vi "md5.vi"(11 "Data in":string) -> (2 "MD5 (16-bytes)":string, 3 "MD5 (Hex String)":string)   [LabVIEW 2021, in "hashlib.lvlib"]
doc: "Calculates the md5 checksum.\n\n[RFC 1321]"
uses:
  hashlib.lvlib
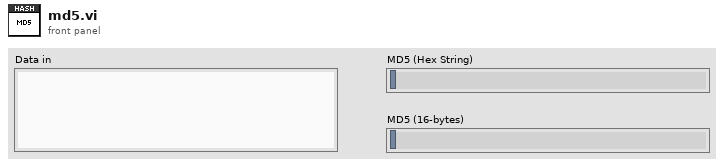
[diagram p1: front panel]
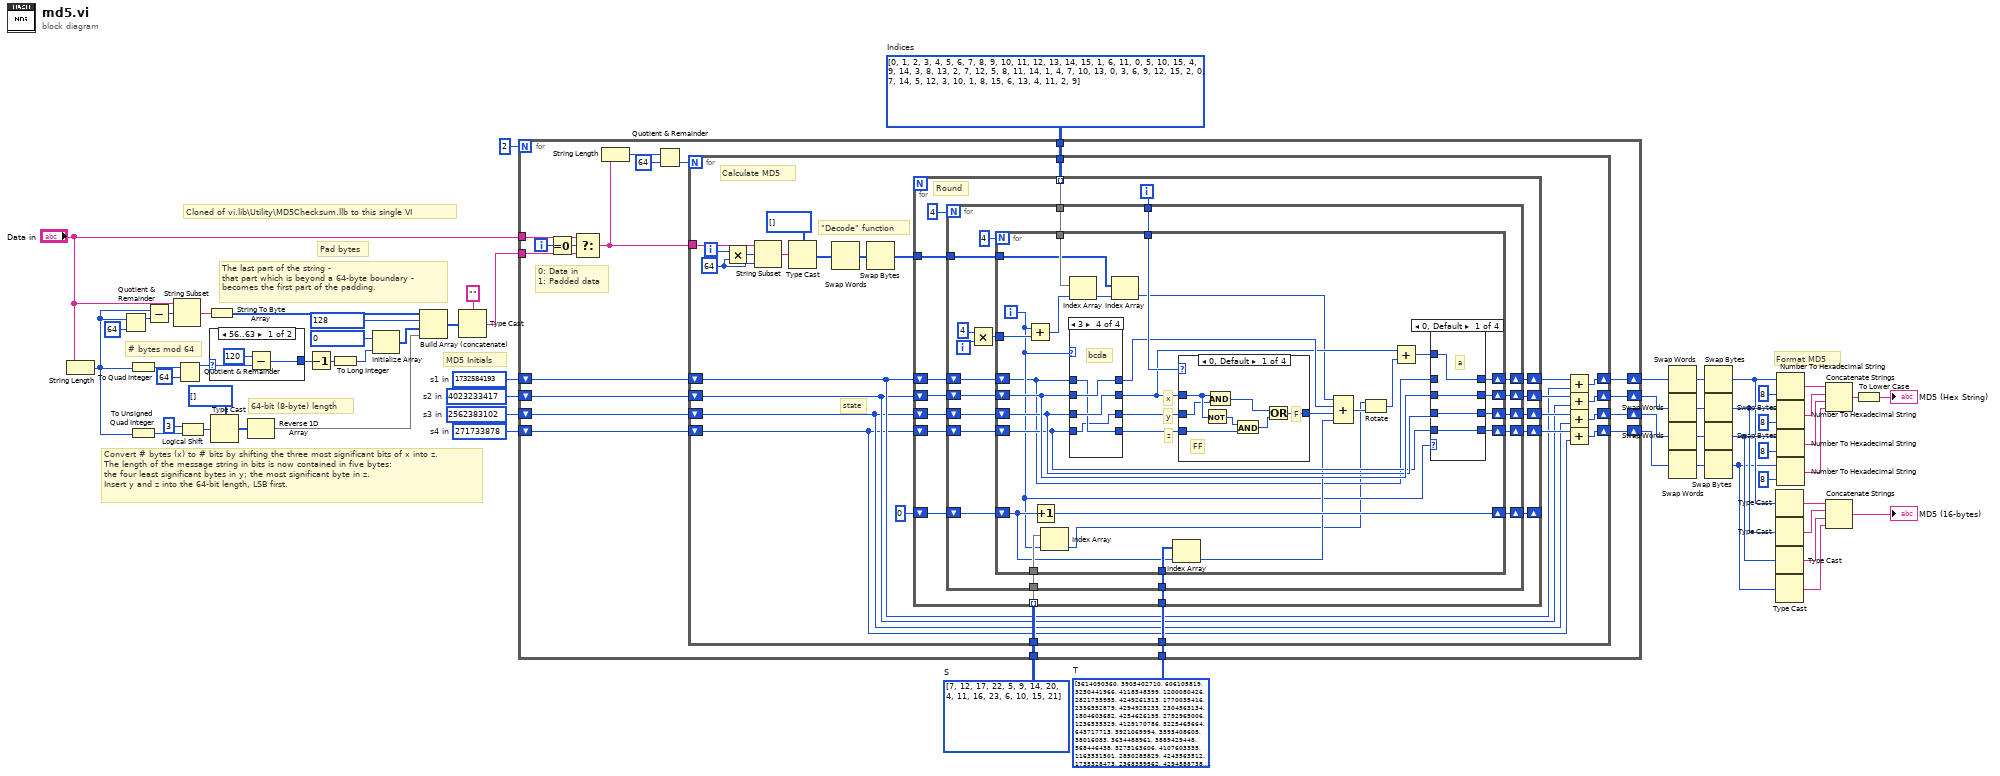
[diagram p0: block diagram]
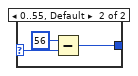
[diagram p2: hidden frame]
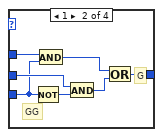
[diagram p3: hidden frame]
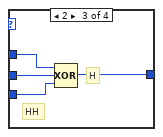
[diagram p4: hidden frame]
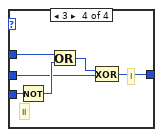
[diagram p5: hidden frame]
diagram:
  w43 = u32 1732584193  # s1 in
  w42 = u32 4023233417  # s2 in
  w41 = u32 2562383102  # s3 in
  w40 = u32 271733878  # s4 in
  w47 = i32[][] [[7, 12, 17, 22], [5, 9, 14, 20], [4, 11, 16, 23], [6, 10, 15, 21]]  # S
  w46 = u32[] [3614090360, 3905402710, 606105819, 3250441966, 4118548399, 1200080426, 2821735955, 4249261313, 1770035416, 2336552879, 4294925233, 2304563134, 1804603682, 4254626195, 2792965006, 1236535329, 4129170786, 3225465664, 643717713, 3921069994, 3593408605, 38016083, 3634488961, 3889429448, 568446438, 3275163606, 4107603335, 1163531501, 2850285829, 4243563512, 1735328473, 2368359562, 4294588738, 2272392833, 1839030562, 4259657740, 2763975236, 1272893353, 4139469664, 3200236656, 681279174, 3936430074, 3572445317, 76029189, 3654602809, 3873151461, 530742520, 3299628645, 4096336452, 1126891415, 2878612391, 4237533241, 1700485571, 2399980690, 4293915773, 2240044497, 1873313359, 4264355552, 2734768916, 1309151649, 4149444226, 3174756917, 718787259, 3951481745]  # T
  w45 = i32[][] [[0, 1, 2, 3, 4, 5, 6, 7, 8, 9, 10, 11, 12, 13, 14, 15], [1, 6, 11, 0, 5, 10, 15, 4, 9, 14, 3, 8, 13, 2, 7, 12], [5, 8, 11, 14, 1, 4, 7, 10, 13, 0, 3, 6, 9, 12, 15, 2], [0, 7, 14, 5, 12, 3, 10, 1, 8, 15, 6, 13, 4, 11, 2, 9]]  # Indices
  # "Cloned of vi.lib\\Utility\\MD5Checksum.llb to this single VI"
  # "Format MD5"
  # "MD5 Initials"
  # "Pad bytes"
  # "The last part of the string - \nthat part which is beyond a 64-byte boundary - \nbecomes the first part of the padding."
  # "64-bit (8-byte) length"
  # "Convert # bytes (x) to # bits by shifting the three most significant bits of x into z.\nThe length of the message string in bits is now contained in five bytes:  \nthe four least significant bytes in y; the most significant byte in z.\nInsert y and z into the 64-bit length, LSB first."
  # "# bytes mod 64"
  n1 = String Length(string="Data in") -> (length=w58:i32)
  n2 = Quotient & Remainder(x=w58, y=64) -> (x-y*floor(x/y)=w57:i32)  [unwired: 1 out]
  n3 = To Quad Integer(1:w58) -> (0:w24:i64)
  n4 = To Unsigned Quad Integer(1:w58) -> (0:w35:u64)
  n5 = Subtract(x=w58, y=w57) -> (x-y=w59:i32)
  n6 = String Subset(string="Data in", offset (0)=w59) -> (substring=w56:string)  [unwired: 1 out]
  n7 = Quotient & Remainder(x=w24, y=i64 64) -> (x-y*floor(x/y)=w33:i64)  [unwired: 1 out]
  n8 = Logical Shift(y=i16 3, x=w35) -> (x << y=w37:u64)
  n9 = String To Byte Array(string=w56) -> (unsigned byte array=w32:u8[])
  n10 = case shown="56..63" w33 {
    selector: w33 -> [w62 w65]
    tunnel: [w61 w64] -> w31
    frame 56..63 {
      n11 = Subtract(x=i64 120, y=w62) -> (x-y=w61:i64)
    }
    frame 0..55, Default {
      n12 = Subtract(x=i64 56, y=w65) -> (x-y=w64:i64)
    }
  }
  n13 = Type Cast(type=u8[] [], x=w37) -> (*(type *) &x=w38:u8[])
  n14 = Reverse 1D Array(array=w38) -> (reversed array=w39:u8[])
  n15 = Decrement(x=w31) -> (x-1=w30:i64)
  n16 = To Long Integer(number=w30) -> (32bit integer=w22:i32)
  n17 = Initialize Array(u8 0, w22) -> (w26:u8[])
  n18 = Build Array (concatenate)(w32, u8 128, w26, w39) -> (w29:u8[])
  n19 = Type Cast(type="", x=w29) -> (*(type *) &x=w52:string)
  n20 = for {
    N: 2 -> [_]
    tunnel: w47 -> [w77]
    tunnel: w46 -> [w76]
    tunnel: w45 -> [w75]
    tunnel: "Data in" -> [w68]
    shift-right: [w78] -> w51
    shift-left: w43 -> [w82]
    shift-right: [w79] -> w50
    shift-left: w42 -> [w83]
    shift-right: [w80] -> w49
    shift-left: w41 -> [w84]
    shift-right: [w81] -> w48
    shift-left: w40 -> [w85]
    tunnel: w52 -> [w67]
    i -> [w71]
    # "0: Data in\n1: Padded data"
    n21 = Equal To 0?(x=w71) -> (x = 0?=w70:bool)
    n22 = Select(t=w68, s=w70, f=w67) -> (s? t:f=w69:string)
    n23 = String Length(string=w69) -> (length=w73:i32)
    n24 = Quotient & Remainder(x=w73, y=64) -> (floor(x/y)=w72:i32)  [unwired: 1 out]
    n25 = for {
      N: w72 -> [_]
      tunnel: w75 -> [w105]
      tunnel: w76 -> [w104]
      tunnel: w77 -> [w103]
      shift-right: [w102] -> w78
      shift-left: w82 -> [w98]
      shift-right: [w101] -> w79
      shift-left: w83 -> [w97]
      shift-right: [w100] -> w80
      shift-left: w84 -> [w96]
      shift-right: [w99] -> w81
      shift-left: w85 -> [w95]
      tunnel: w69 -> [w93]
      i -> [w94]
      w86 = 64 ("y")
      # "Calculate MD5"
      # "\"Decode\" function"
      # "state"
      n26 = Multiply(x=w94, y=w86) -> (x*y=w90:i32)
      n27 = String Subset(string=w93, offset (0)=w90, length (rest)=w86) -> (substring=w92:string)
      n28 = Type Cast(type=u32[] [], x=w92) -> (*(type *) &x=w88:u32[])
      n29 = Swap Words(1:w88) -> (0:w89:u32[])
      n30 = Swap Bytes(anything=w89) -> (byte swapped=w87:u32[])
      n31 = for {
        shift-right: [w121] -> w107
        shift-left: w98 -> [w122]
        shift-right: [w120] -> w108
        shift-left: w97 -> [w123]
        shift-right: [w119] -> w109
        shift-left: w96 -> [w124]
        shift-right: [w118] -> w110
        shift-left: w95 -> [w125]
        tunnel: w105 -> [w117] mode=indexing
        tunnel: w103 -> [w116] mode=indexing
        tunnel: w87 -> [w115]
        shift-right: [w112] -> _
        shift-left: 0 -> [w113]
        tunnel: w104 -> [w111]
        i -> [w126]
        # "Round"
        n32 = for {
          N: 4 -> [_]
          tunnel: w126 -> [w145]
          shift-right: [w138] -> w118
          shift-left: w125 -> [w139]
          shift-right: [w137] -> w119
          shift-left: w124 -> [w140]
          shift-right: [w143] -> w120
          shift-left: w123 -> [w141]
          shift-right: [w144] -> w121
          shift-left: w122 -> [w142]
          tunnel: w117 -> [w136]
          tunnel: w116 -> [w135]
          tunnel: w115 -> [w131]
          shift-right: [w128] -> w112
          shift-left: w113 -> [w129]
          tunnel: w111 -> [w127]
          i -> [w134]
          n33 = Multiply(x=4, y=w134) -> (x*y=w132:i32)
          n34 = for {
            N: 4 -> [_]
            tunnel: w145 -> [w157]
            shift-right: [w167] -> w138
            shift-left: w139 -> [w162]
            shift-right: [w166] -> w137
            shift-left: w140 -> [w163]
            shift-right: [w165] -> w143
            shift-left: w141 -> [w164]
            shift-right: [w168] -> w144
            shift-left: w142 -> [w148]
            tunnel: w136 -> [w175]
            tunnel: w135 -> [w174]
            tunnel: w132 -> [w161]
            tunnel: w131 -> [w171]
            shift-right: [w158] -> w128
            shift-left: w129 -> [w159]
            tunnel: w127 -> [w160]
            i -> [w149]
            # "z"
            # "y"
            # "x"
            n35 = Add(x=w149, y=w161) -> (x+y=w173:i32)
            n36 = Increment(x=w159) -> (x+1=w158:i32)
            n37 = Index Array(array=w174, index=w149) -> (element=w147:i32)
            n38 = Index Array(array=w175, index=w173) -> (element=w172:i32)
            n39 = case shown="3" w149 {
              tunnel: w148 -> [w219 w222 w225 w229]
              tunnel: w164 -> [w218 w221 w224 w231]
              tunnel: w163 -> [w217 w220 w227 w230]
              tunnel: w162 -> [w216 w223 w226 w228]
              tunnel: [w219 w223 w227 w231] -> w152
              tunnel: [w218 w222 w226 w230] -> w151
              tunnel: [w217 w221 w225 w228] -> w170
              tunnel: [w216 w220 w224 w229] -> w169
              frame 0, Default {
                # "abcd"
              }
              frame 1 {
                # "dabc"
              }
              frame 2 {
                # "cdab"
              }
              frame 3 {
                # "bcda"
              }
            }
            n40 = Index Array(array=w171, index=w172) -> (element=w146:u32)
            n41 = Index Array(array=w160, index=w159) -> (element=w154:u32)
            n42 = case shown="0, Default" w157 {
              tunnel: w151 -> [w179 w185 w192 w196]
              tunnel: w170 -> [w178 w184 w193 w195]
              tunnel: w169 -> [w177 w183 w191 w194]
              tunnel: [w176 w186 w190 w197] -> w153
              frame 0, Default {
                # "FF"
                # "F"
                n43 = Not(x=w179) -> (.not. x?=w182:u32)
                n44 = And(x=w179, y=w178) -> (x .and. y?=w181:u32)
                n45 = And(x=w182, y=w177) -> (x .and. y?=w180:u32)
                n46 = Or(x=w181, y=w180) -> (x .or. y?=w176:u32)
              }
              frame 1 {
                # "GG"
                # "G"
                n47 = Not(x=w183) -> (.not. x?=w187:u32)
                n48 = And(x=w185, y=w183) -> (x .and. y?=w188:u32)
                n49 = And(x=w184, y=w187) -> (x .and. y?=w189:u32)
                n50 = Or(x=w188, y=w189) -> (x .or. y?=w186:u32)
              }
              frame 2 {
                # "H"
                # "HH"
                n51 = Compound Arithmetic op=XOR(w192, w193, w191) -> (w190:u32)
              }
              frame 3 {
                # "I"
                # "II"
                n52 = Not(x=w194) -> (.not. x?=w199:u32)
                n53 = Or(x=w196, y=w199) -> (x .or. y?=w198:u32)
                n54 = Exclusive Or(1:w195, 2:w198) -> (0:w197:u32)
              }
            }
            n55 = Compound Arithmetic op=ADD(w146, w152, w153, w154) -> (w156:u32)
            n56 = Rotate(1:w156, 2:w147) -> (0:w150:u32)
            n57 = Add(x=w151, y=w150) -> (x+y=w155:u32)
            n58 = case shown="0, Default" w149 {
              tunnel: w155 -> [w203 w207 w211 w215]
              tunnel: [w203 w206 w210 w214] -> w168
              tunnel: [w200 w207 w208 w212] -> w167
              tunnel: [w201 w204 w211 w213] -> w166
              tunnel: [w202 w205 w209 w215] -> w165
              tunnel: w148 -> [_ w206 w210 w214]
              tunnel: w164 -> [w202 w205 w209 _]
              tunnel: w163 -> [w201 w204 _ w213]
              tunnel: w162 -> [w200 _ w208 w212]
              frame 0, Default {
                # "a"
              }
              frame 1 {
                # "d"
              }
              frame 2 {
                # "c"
              }
              frame 3 {
                # "b"
              }
            }
          }
        }
      }
      n59 = Add(x=w107, y=w98) -> (x+y=w102:u32)
      n60 = Add(x=w108, y=w97) -> (x+y=w101:u32)
      n61 = Add(x=w109, y=w96) -> (x+y=w100:u32)
      n62 = Add(x=w110, y=w95) -> (x+y=w99:u32)
    }
  }
  n63 = Swap Words(1:w51) -> (0:w2:u32)
  n64 = Swap Words(1:w50) -> (0:w3:u32)
  n65 = Swap Words(1:w49) -> (0:w6:u32)
  n66 = Swap Words(1:w48) -> (0:w7:u32)
  n67 = Swap Bytes(anything=w2) -> (byte swapped=w15:u32)
  n68 = Swap Bytes(anything=w3) -> (byte swapped=w16:u32)
  n69 = Swap Bytes(anything=w6) -> (byte swapped=w17:u32)
  n70 = Swap Bytes(anything=w7) -> (byte swapped=w14:u32)
  n71 = Type Cast(x=w15) -> (*(type *) &x=w18:string)  [unwired: 1 in]
  n72 = Type Cast(x=w16) -> (*(type *) &x=w19:string)  [unwired: 1 in]
  n73 = Type Cast(x=w17) -> (*(type *) &x=w20:string)  [unwired: 1 in]
  n74 = Type Cast(x=w14) -> (*(type *) &x=w21:string)  [unwired: 1 in]
  n75 = Number To Hexadecimal String(1:i16 8 ("width (-)"), 2:w15) -> (0:w9:string)
  n76 = Number To Hexadecimal String(1:i16 8 ("width (-)"), 2:w16) -> (0:w10:string)
  n77 = Number To Hexadecimal String(1:i16 8 ("width (-)"), 2:w17) -> (0:w11:string)
  n78 = Number To Hexadecimal String(1:i16 8 ("width (-)"), 2:w14) -> (0:w12:string)
  n79 = Concatenate Strings(w9, w10, w11, w12) -> (w13:string)
  n80 = Concatenate Strings(w18, w19, w20, w21) -> (→"MD5 (16-bytes)":string)
  n81 = To Lower Case(string=w13) -> (all lower case string=→"MD5 (Hex String)":string)
